vi "CalcOneTap.vi"(11 "wavform file":path) -> (0 "Settings":T1={"Name of test"="", "Date"=timestamp(0 s since 1904-01-01), "Location"="", "Template"="", "Soundcard"="", "resolution"=0, "Sampling rate"=0, "Ch1 Gain "=0.0, "Ch2 Gain"=0.0, "Sample time (s)"=0.0, "Pre-trigger (s)"=0.0, "Hammer Threshold"=0.0, "Positions"=0, "Taps/Position"=0, "Set Names"="", "Freq resolution"=0.0, "Hammer cutoff"=0.0, "Mic cutoff"=0.0, "Double bounce "=0.0, "Hammer Cal"=0.0, "dB Offset"=0.0, "Accel Cal"=0.0, "Vibrometer Cal"=0.0, "Mic Cal"=0.0, "Output"=0, "Voltage Cal"=0.0, "Vibrometer Port"="", "Range"=0, "High Pass"=0, "Bandwidth"=0, "X Range"=[], "Y Range"=[], "dB Spread"=0.0, "Trigger"=0, "Ch_1"=0, "Ch_2"=0, "flip?"=FALSE, "60Hz"=FALSE, "Time offset"=0.0, "Piezo Cal"=1.0, "Default Notes"=""} {"Ch_2" min=1 step=1; "Ch_1" min=1 max=100 step=1; "Trigger" items=["Hammer (force)", "Self-tap", "Spacebar"]; "Bandwidth" items=["1 kHz"=1, "5 kHz"=5, "10 kHz"=10, "25 kHz"=25, "50 kHz"=50, "100 kHz"=100]; "High Pass" items=["Off", "13 Hz", "104 Hz"]; "Range" items=["10 mm/s"=1, "20 mm/s"=2, "50 mm/s"=5, "100 mm/s"=10, "200 mm/s"=20, "500 mm/s"=50, "1 m/s"=100, "2 m/s"=200]; "Output" items=["Accelerometer", "Speed (from acceleration)", "Microphone", "Vibrometer", "Piezo"]; "Voltage Cal" format="%#_13g"; "Ch2 Gain" format="%#_13g"; "Ch1 Gain" format="%#_13g"; "Double bounce" min=0.0; "Mic cutoff" min=0.0 format="%#_4g"; "Hammer cutoff" min=0.0 format="%#_4g"; "Freq resolution" min=0.0; "Pre-trigger (s)" format="%#_13g"; "Date" format="%<%H:%M\n%d/%m/%y>T"; "resolution" items=["16 bit"=16, "24 bit"=24, "32 bit"=32]; "Sampling rate" items=["22050 samp/s"=22050, "44100 samp/s"=44100, "48000 samp/s"=48000]}, 1 "Complex FRF":cluster{dbl, "df":dbl, cdb[]}, 2 "info":cluster{"Sampling rate":dbl, "npts":dbl}, 3 "FRF":cluster{dbl, "dt":dbl, "Y":dbl[]}(graph))   [LabVIEW 2022 SP3]
uses:
  PreferencesControl.ctl
panel:
  # "Hz"
  # "dB"
  # "dB"
  # "sec"
  # "sec"
  # "mV/Pa"
  # "mV/m/s2"
  # "mV/mm/s"
  # "V/N"
  # "sec"
  # "sec"
  # "mV/N"
  # "a.u."
  # "a.u."
  # "sec"
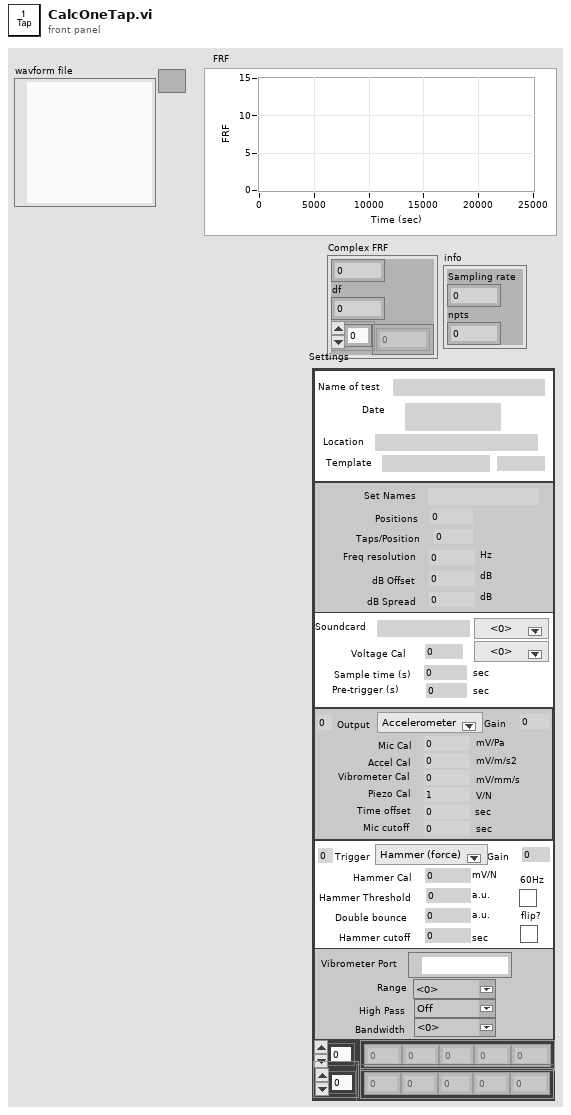
[diagram p1: front panel]
types:
  T1 = typedef "PreferencesControl.ctl" = cluster{"Name of test":string, "Date":timestamp, "Location":string, "Template":string, "Soundcard":string, "resolution":u16, "Sampling rate":u16, "Ch1 Gain ":dbl, "Ch2 Gain":dbl, "Sample time (s)":dbl, "Pre-trigger (s)":dbl, "Hammer Threshold":dbl, "Positions":i16, "Taps/Position":i16, "Set Names":string, "Freq resolution":dbl, "Hammer cutoff":dbl, "Mic cutoff":dbl, "Double bounce ":dbl, "Hammer Cal":dbl, "dB Offset":dbl, "Accel Cal":dbl, "Vibrometer Cal":dbl, "Mic Cal":dbl, "Output":u16, "Voltage Cal":dbl, "Vibrometer Port":refnum<visa-resource-name>, "Range":u16, "High Pass":u16, "Bandwidth":u16, "X Range":cluster{"Minimum":dbl, "Maximum":dbl, "Increment":dbl, "Minor Increment":dbl, "Start":dbl}[], "Y Range":cluster{"Minimum":dbl, "Maximum":dbl, "Increment":dbl, "Minor Increment":dbl, "Start":dbl}[], "dB Spread":dbl, "Trigger":u16, "Ch_1":u8, "Ch_2":u8, "flip?":bool, "60Hz":bool, "Time offset":dbl, "Piezo Cal":dbl, "Default Notes":string}
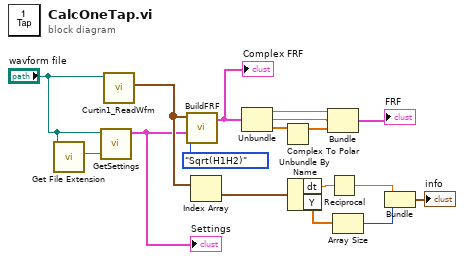
[diagram p0: block diagram]
diagram:
  n1 = call <vilib>:"Get File Extension.vi"("file"="wavform file") -> ("lowercase file extension"=w1:string)  [unwired: 6 in, 4 out]
  n2 = call "GetSettings.vi"("lowercase file extension"=w1, "wavform file"="wavform file") -> ("Settings"=w9:T1)  [unwired: 8 in, 1 out]
  "Settings" <- w9
  n3 = call "Curtin1_ReadWfm.vi"("appended path"="wavform file") -> ("all waveforms in record"=w10:waveform(dbl)[])  [unwired: 9 in, 1 out]
  n4 = call "BuildFRF.vi"("Method"=enum16{"Sqrt(H1H2)", "H1", "H2"}."Sqrt(H1H2)", "Settings"=w9, "Data In"=w10) -> ("Complex FRF"=w12:cluster{"t0":dbl, "dt":dbl, "Y":cdb[]})  [unwired: 3 in, 5 out]
  "Complex FRF" <- w12
  n5 = Index Array(array=w10) -> (element=w8:waveform(dbl))  [unwired: 1 in]
  n6 = Unbundle(w12) -> ("t0"=w14:dbl, "dt"=w13:dbl, "Y"=w17:cdb[])
  n7 = Complex To Polar(r * e^(i*theta)=w17) -> (r=w16:dbl[])  [unwired: 1 out]
  n8 = Unbundle By Name(w8) -> ("dt"=w7:dbl, "Y"=w5:dbl[])
  n9 = Bundle("t0"=w14, "dt"=w13, w16) -> (→"FRF":cluster{"t0":dbl, "dt":dbl, dbl[]})  [unwired: 1 in]
  n10 = Reciprocal(x=w7) -> (1/x=w6:dbl)
  n11 = Array Size(array=w5) -> (size(s)=w4:i32)
  n12 = Bundle(w6, w4) -> (→"info":cluster{dbl, i32})  [unwired: 1 in]
